vi "Support_ClearError.vi"(2 "code":i32, 5 "error in (no error)":errorcluster) -> (16 "Cleared?":bool, 19 "error out":errorcluster)   [LabVIEW 2020]
doc: "Use this VI to ignore errors with a certain code."
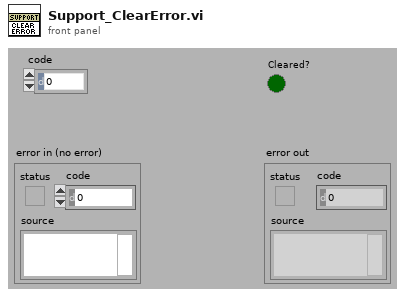
[diagram p1: front panel]
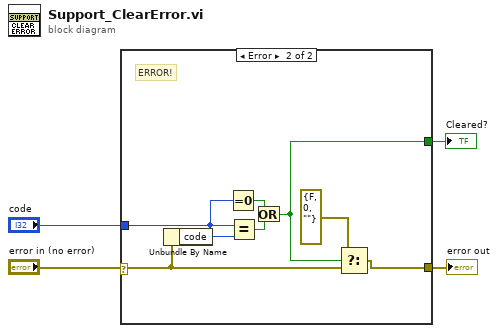
[diagram p0: block diagram]
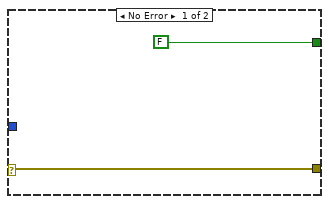
[diagram p2: hidden frame]
diagram:
  n1 = case shown="Error" "error in (no error)" {
    selector: "error in (no error)" -> [w5 w11]
    tunnel: [w5 w13] -> w4
    tunnel: "code" -> [_ w10]
    tunnel: [FALSE w7] -> w2
    frame No Error {
    }
    frame Error {
      # "ERROR!"
      n2 = Unbundle By Name(w11) -> ("code"=w14:i32)
      n3 = Equal To 0?(x=w10) -> (x = 0?=w9:bool)
      n4 = Equal?(x=w10, y=w14) -> (x = y?=w8:bool)
      n5 = Or(x=w9, y=w8) -> (x .or. y?=w7:bool)
      n6 = Select(t=errorcluster {"status"=FALSE, "code"=0, "source"=""}, s=w7, f=w11) -> (s? t:f=w13:errorcluster)
    }
  }
  "error out" <- w4
  "Cleared?" <- w2
